vi "createFPGA.vi"(8 "error in (no error)":errorcluster, 11 "Boot in":refnum<class "Boot.lvclass">) -> (0 "error out":errorcluster, 2 "FPGA":refnum<class "FPGA.lvclass">, 3 "Boot out":refnum<class "Boot.lvclass">)   [LabVIEW 2016, in "Boot.lvclass"]
uses:
  Boot.lvclass
  Resources/FPGA/FPGA.lvclass
  Boot.lvclass/Boot.ctl
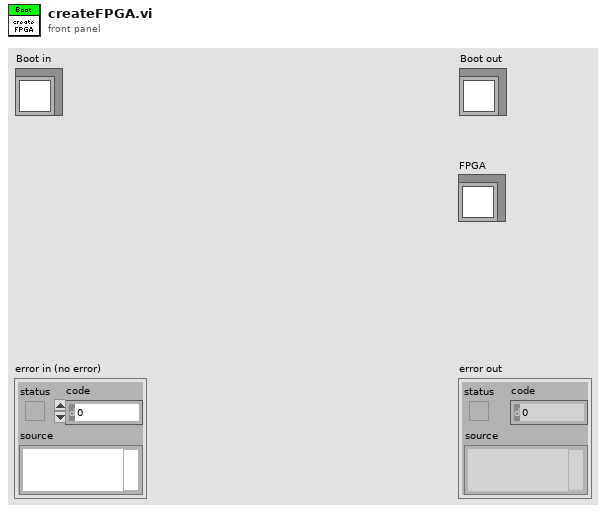
[diagram p1: front panel]
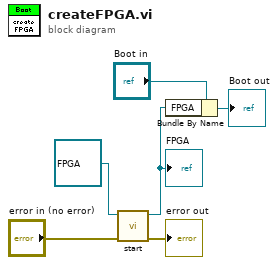
[diagram p0: block diagram]
diagram:
  n1 = call "start.vi"("error in (no error)"="error in (no error)", "FPGA in"=refnum<class "FPGA.lvclass"> refnum ("FPGA.lvclass")) -> ("error out"=→"error out":errorcluster, "FPGA out"=w3:refnum<class "FPGA.lvclass">)  [unwired: 8 in]
  "FPGA" <- w3
  n2 = Bundle By Name(cluster="Boot in", "FPGA"=w3) -> (→"Boot out":refnum<class "Boot.lvclass">)
